vi "Actor Core.vi"(8 "error in":errorcluster, 11 "Example Actor in":refnum<class "Example Actor.lvclass">) -> (0 "error out":errorcluster, 3 "Actor out":refnum<class "Actor.lvclass">)   [LabVIEW 2023, in "Example Iterator NR Actor Implicit Iteration.lvlib" / "Example Actor.lvclass"]
doc: "(<B>Filename</B>: Actor Framework.lvlib:Actor.lvclass:Actor Core.vi)\n\nReceives messages to the actor, reacts to them, and initiates any error handling that may shut the actor down.\n\nDescendant classes may override this VI to append parallel tasks for the actor to complete while it handles messages. Overrides use the Call Parent Method node."
uses:
  Example Actor.lvclass
  <vilib>/ActorFramework/Actor/Actor.lvclass
  Iterator Settings.ctl
  Abstract Iterator Actor/Active Stop Conditions.ctl
  Abstract Iterator Actor/Stop Reason.ctl
  Iterator NR Actor/Iterator NR Actor Folder/Iterator NR Actor.lvclass
  Example Actor.lvclass/Example Actor.ctl
  <vilib>/ActorFramework/Actor/Actor.lvclass/Actor.ctl
  <vilib>/ActorFramework/Message Enqueuer/Message Enqueuer.lvclass/Message Enqueuer.ctl
  Example Actor Messages/Iterate Reply Msg/Iteration Msg.lvclass
  Abstract Iterator Actor/Iterator Settings.ctl
  <vilib>/ActorFramework/Message/Message.lvclass
  Iterator Actor/Iterator Actor Abstract Messages/Iterator Report Iterations End Msg/Iterator Report Iterations End Msg.lvclass
  <vilib>/ActorFramework/Message Enqueuer/Message Priority.ctl
  Example Actor Messages/Pre Iterate Reply Msg/Pre Iteration Msg.lvclass
  Example Actor Messages/Post Iterate Reply Msg/Post Iteration Msg.lvclass
  Example Actor Messages/Update Error Msg/Update Error Msg.lvclass
  <vilib>/ActorFramework/Message Enqueuer/Init from Existing Queue.vi
  <vilib>/ActorFramework/Message Enqueuer/Enqueue.vi
  <vilib>/ActorFramework/Stop Msg/Stop Msg.lvclass
  <vilib>/ActorFramework/Message Priority Queue/Priority Enqueue.vi
  <vilib>/ActorFramework/Message Enqueuer/Message Enqueuer.lvclass
  Example Actor Messages/Write Ready for iterations Msg/Write Ready for iterations Msg.lvclass
  Iterator Actor/Iterator Actor Messages/Write Settings Msg/Write Settings Msg.lvclass
  Iterator Actor/Iterator Actor Messages/Start Iterations Msg/Start Iterations Msg.lvclass
  Iterator Actor/Iterator Actor Messages/Stop Iterations Msg/Stop Iterations Msg.lvclass
  C:/Program Files/National Instruments/LabVIEW 2023/vi.lib/ActorFramework/Actor/Actor.lvclass
  C:/Projects/Iterator Actor/Examples/Example Iterator NR Actor Implicit Iteration/Example Actor/Example Actor.lvclass
  Abstract Iterator Actor/Abstract Iterator Actor.lvclass
  C:/Projects/Iterator Actor/Abstract Iterator Actor/Abstract Iterator Actor.lvclass
  C:/Program Files/National Instruments/LabVIEW 2023/vi.lib/LS Instruments AG/Async Methods Actor/Async Methods Actor/Async Methods Actor/Async Methods Actor.lvclass
  C:/Projects/Iterator Actor/Iterator NR Actor/Iterator NR Actor Folder/Iterator NR Actor.lvclass
  C:/Projects/Iterator Actor/Iterator NR Actor/Iterator NR Actor Messages/Iteration Msg/Abstract Iteration Msg.lvclass
  C:/Program Files/National Instruments/LabVIEW 2023/vi.lib/ActorFramework/Message/Message.lvclass
  C:/Projects/Iterator Actor/Examples/Example Iterator NR Actor Implicit Iteration/Example Actor Messages/Iterate Reply Msg/Iteration Msg.lvclass
  C:/Projects/Iterator Actor/Examples/Example Iterator NR Actor Implicit Iteration/Example Actor Messages/Pre Iterate Reply Msg/Pre Iteration Msg.lvclass
  C:/Projects/Iterator Actor/Examples/Example Iterator NR Actor Implicit Iteration/Example Actor Messages/Post Iterate Reply Msg/Post Iteration Msg.lvclass
  C:/Projects/Iterator Actor/Iterator Actor/Iterator Actor Abstract Messages/Iterator Report Iterations End Msg/Iterator Report Iterations End Msg.lvclass
  C:/Projects/Iterator Actor/Examples/Example Iterator NR Actor Implicit Iteration/Example Actor Messages/Update Error Msg/Update Error Msg.lvclass
panel:
  out "Stop Reason":T1
  in  "Receive report":bool=TRUE
  in  "Do post-iterations":bool=TRUE
  in  "Do pre-iterations":bool=TRUE
  out "Iterator error":errorcluster
  in  "User Settings":T2={"Prepare timeout (ms)"=1000, "Iterate timeout (ms)"=1000, "Conclude timeout (ms)"=1000, "Iterate period (ms)"=1000, "Active Stop Conditions"={"Number of Iterations"=FALSE, "Time Elapsed"=FALSE, "Iteration Result"=FALSE}, "Iterations"=5, "Time before stop (ms)"=200}
  out "Post Iterate":bool
  out "Pre Iterate":bool
  in  "exit":bool
  out "Iterate":bool
  in  "stop iterations":bool
  in  "start iterations":bool
  in  "Ready for iterations":bool=TRUE
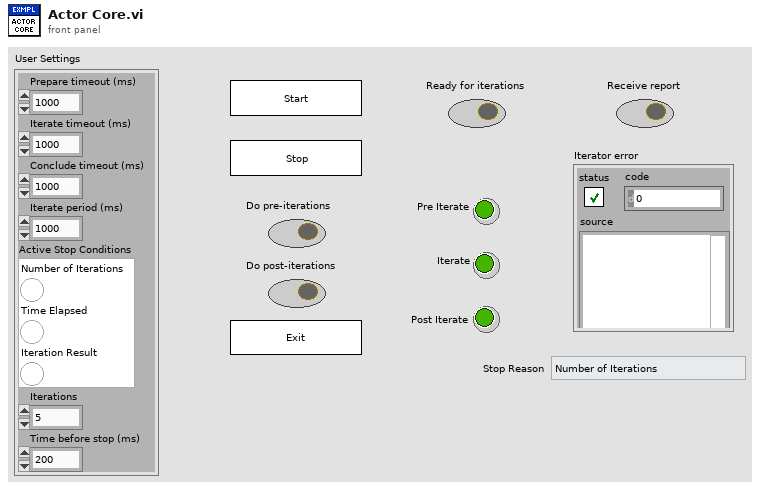
[diagram p1: front panel]
types:
  T1 = typedef "Iterator Actor.lvlib/Abstract Iterator Actor.lvclass/Stop Reason.ctl" = enum16{"Number of Iterations", "Time Elapsed", "Stopped Internally", "Stopped Externally"}
  T2 = typedef "Example Iterator NR Actor Implicit Iteration.lvlib/Example Actor.lvclass/Iterator Settings.ctl" = cluster{"Prepare timeout (ms)":i32, "Iterate timeout (ms)":i32, "Conclude timeout (ms)":i32, "Iterate period (ms)":i32, "Active Stop Conditions":T3, "Iterations":i32, "Time before stop (ms)":i32}
  T3 = typedef "Iterator Actor.lvlib/Abstract Iterator Actor.lvclass/Active Stop Conditions.ctl" = cluster{"Number of Iterations":bool, "Time Elapsed":bool, "Iteration Result":bool}
  T4 = typedef "Iterator Actor.lvlib/Abstract Iterator Actor.lvclass/Iterator Settings.ctl" = cluster{"Prepare timeout (ms)":i32, "Iterate timeout (ms)":i32, "Conclude timeout (ms)":i32, "Iterate period (ms)":i32, "Number of iterations":i32, "Time before stop (ms)":i32, "Active Stop Conditions":T3, "Prepare Msg":refnum<class "Message.lvclass">, "Iterate Msg":refnum<class "Message.lvclass">, "Conclude Msg":refnum<class "Message.lvclass">, "Iterations End Report":refnum<class "Iterator Report Iterations End Msg.lvclass">, "Message Priority (Normal)":T5}
  T5 = typedef "Actor Framework.lvlib/Message Enqueuer.lvclass/Message Priority.ctl" = enum16{"Low", "Normal", "High"}
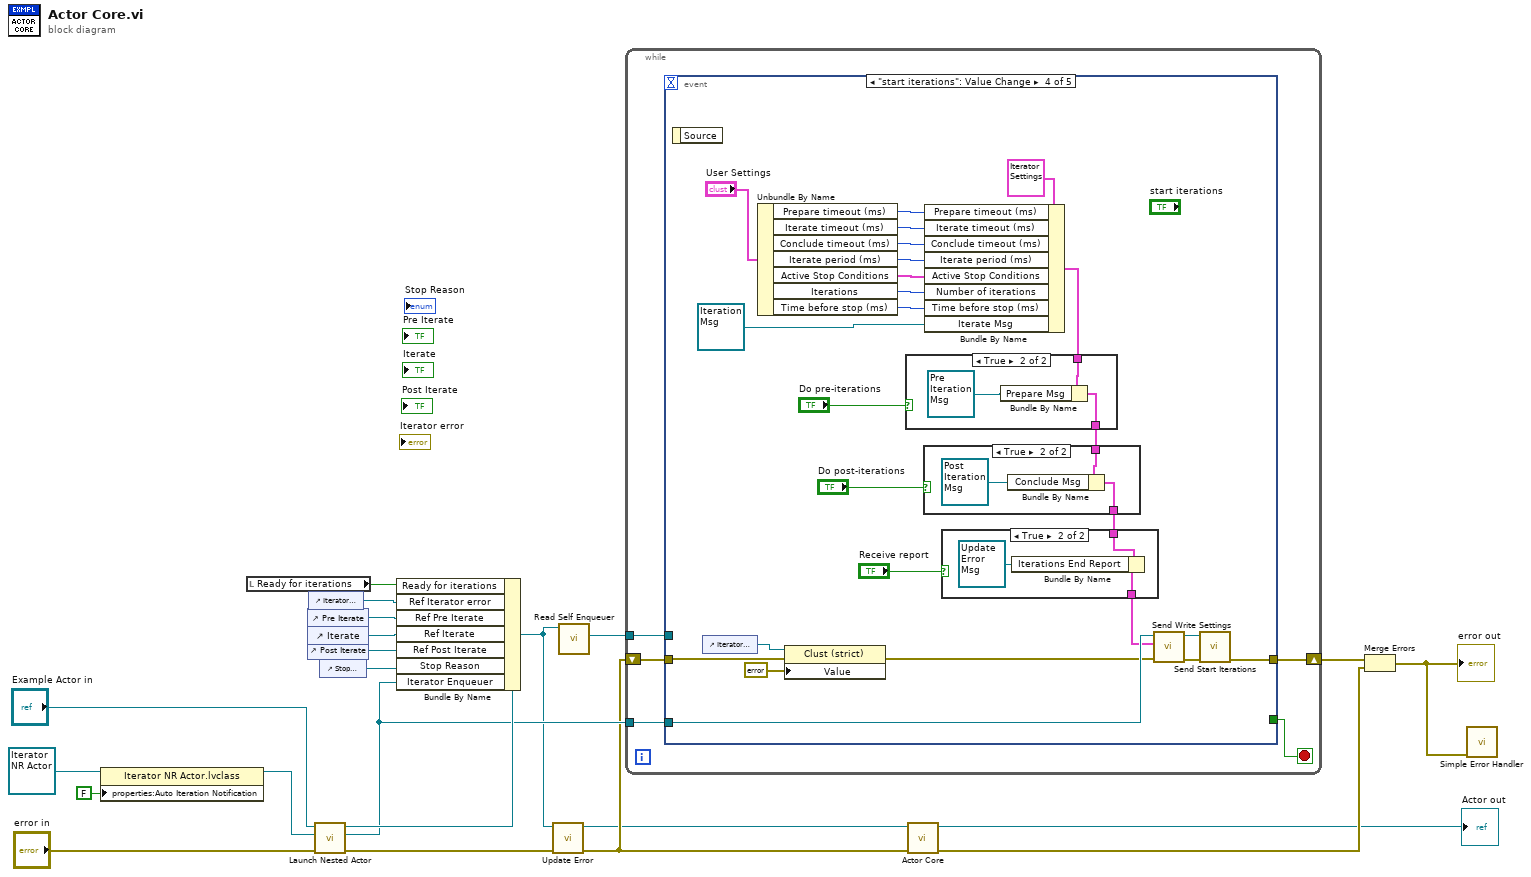
[diagram p0: block diagram]
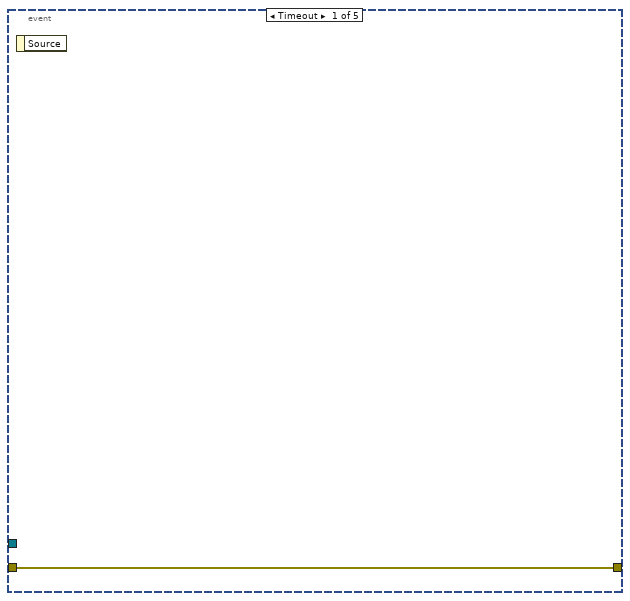
[diagram p2: hidden frame]
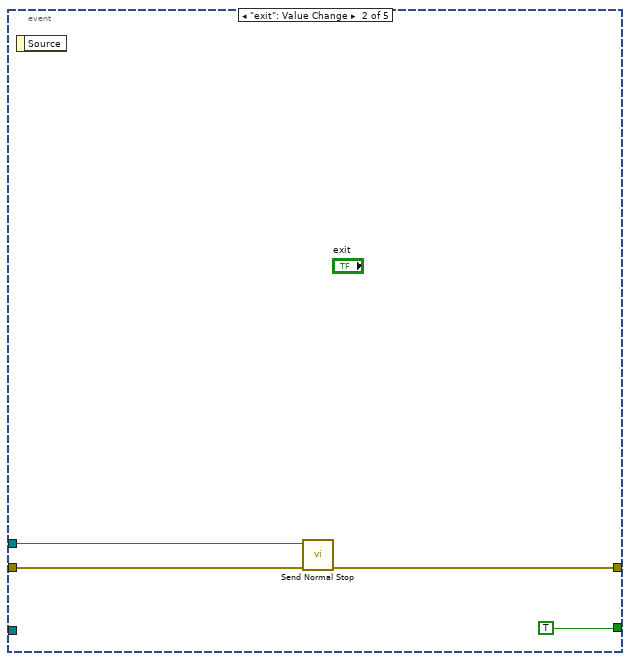
[diagram p3: hidden frame]
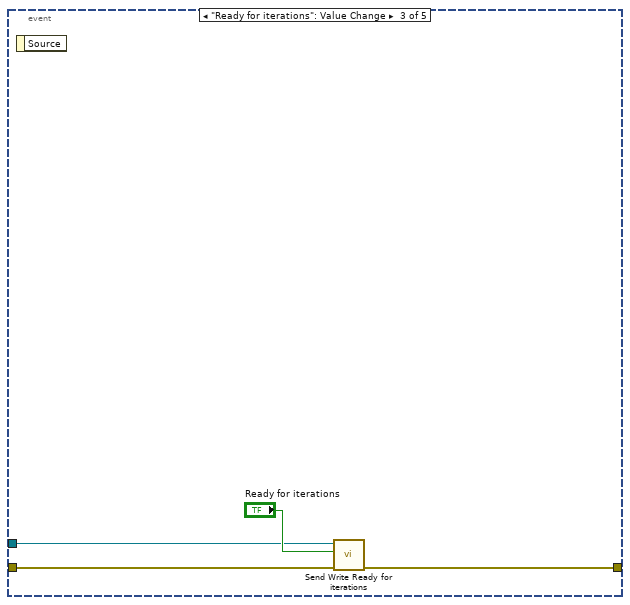
[diagram p4: hidden frame]
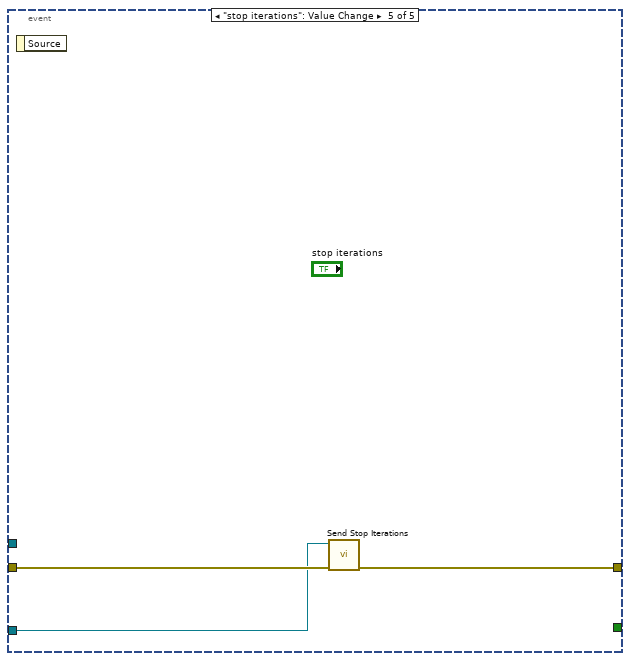
[diagram p8: hidden frame]
diagram:
  n1 = property class="Iterator NR Actor.lvclass"(reference=refnum<class "Iterator NR Actor.lvclass"> refnum ("Iterator Actor 2.lvlib:Iterator Actor 2.lvclass"), "properties:Auto Iteration Notification"=FALSE ("Auto Iteration Notification")) -> (reference out=w2:refnum<class "Iterator NR Actor.lvclass">)  [unwired: 1 in, 1 out]
  n2 = local read "Ready for iterations"() -> (w13:bool)
  n3 = control-ref of="Pre Iterate"() -> (w18:refnum<vi>)
  n4 = control-ref of="Iterate"() -> (w17:refnum<vi>)
  n5 = control-ref of="Post Iterate"() -> (w16:refnum<vi>)
  n6 = control-ref of="Iterator error"() -> (w11:refnum<vi>)
  n7 = call <vilib>:"Launch Nested Actor.vi"("error in (no error)"="error in", "Nested Actor"=w2, "Caller Actor in"="Example Actor in") -> ("error out"=w10:errorcluster, "Nested Actor's Enqueuer"=w14:refnum<class "Message Enqueuer.lvclass">, "Caller Actor out"=w15:refnum<class "Example Actor.lvclass">)  [unwired: 6 in]
  n8 = control-ref of="Stop Reason"() -> (w6:refnum<vi>)
  n9 = Bundle By Name(cluster=w15, "Ready for iterations"=w13, "Ref Iterator error"=w11, "Ref Pre Iterate"=w18, "Ref Iterate"=w17, "Ref Post Iterate"=w16, "Stop Reason"=w6, "Iterator Enqueuer"=w14) -> (w8:refnum<class "Example Actor.lvclass">)
  n10 = call "Update Error.vi"("error in (no error)"=w10, "Example Actor in"=w8) -> ("error out"=w9:errorcluster, "Example Actor out"=w7:refnum<class "Example Actor.lvclass">)  [unwired: 8 in]
  n11 = call <vilib>:"Read Self Enqueuer.vi"("Actor"=w8) -> ("Self Enqueuer"=w22:refnum<class "Message Enqueuer.lvclass">)  [unwired: 10 in]
  n12 = while {
    tunnel: w22 -> [w27]
    shift-right: [w26] -> w21
    shift-left: w9 -> [w25]
    tunnel: w14 -> [w23]
    stop <- w24 stop-if-true
    n13 = event shown="[3] \"start iterations\": Value Change" {
      selector: _ -> [_ _ _ _ _]
      dyn-events: _ -> [_ _ _ _ _]
      timeout: _ -> [_ _ _ _ _]
      tunnel: w27 -> [_ w32 w33 _ _]
      tunnel: [w28 w31 w34 w46 w75] -> w26
      tunnel: w25 -> [w28 w30 w36 w49 w76]
      tunnel: [_ TRUE _ _ _] -> w24
      tunnel: w23 -> [_ _ _ w60 w74]
      event Timeout {
        n14 = event-data() -> ()  [unwired: 1 in, 1 out]
      }
      event "exit": Value Change {
        n15 = event-data() -> ()  [unwired: 1 in, 1 out]
        n16 = call <vilib>:"Send Normal Stop.vi"("error in (no error)"=w30, "Message Enqueuer"=w32) -> ("error out"=w31:errorcluster)  [unwired: 9 in]
      }
      event "Ready for iterations": Value Change {
        n17 = event-data() -> ()  [unwired: 1 in, 1 out]
        n18 = call "Send Write Ready for iterations.vi"("error in (no error)"=w36, "Ready for iterations"="Ready for iterations", "Message Enqueuer in"=w33) -> ("error out"=w34:errorcluster)  [unwired: 7 in, 1 out]
      }
      event "start iterations": Value Change {
        n19 = event-data() -> ()  [unwired: 1 in, 1 out]
        n20 = control-ref of="Iterator error"() -> (w48:refnum<vi>)
        n21 = Unbundle By Name("User Settings") -> ("Prepare timeout (ms)"=w53:i32, "Iterate timeout (ms)"=w54:i32, "Conclude timeout (ms)"=w55:i32, "Iterate period (ms)"=w56:i32, "Active Stop Conditions"=w50:T3, "Iterations"=w51:i32, "Time before stop (ms)"=w52:i32)
        n22 = property class="Clust (strict)"(reference=w48, error in=w49, "Value"=errorcluster {"status"=FALSE, "code"=0, "source"=""}) -> (error out=w44:errorcluster)  [unwired: 1 out]
        n23 = Bundle By Name(cluster=T4 {"Prepare timeout (ms)"=0, "Iterate timeout (ms)"=0, "Conclude timeout (ms)"=0, "Iterate period (ms)"=0, "Number of iterations"=0, "Time before stop (ms)"=0, "Active Stop Conditions"={"Number of Iterations"=FALSE, "Time Elapsed"=FALSE, "Iteration Result"=FALSE}, "Prepare Msg"=refnum, "Iterate Msg"=refnum, "Conclude Msg"=refnum, "Iterations End Report"=refnum, "Message Priority (Normal)"=enum."Normal"} ("Iterator Settings"), "Prepare timeout (ms)"=w53, "Iterate timeout (ms)"=w54, "Conclude timeout (ms)"=w55, "Iterate period (ms)"=w56, "Active Stop Conditions"=w50, "Number of iterations"=w51, "Time before stop (ms)"=w52, "Iterate Msg"=refnum<class "Iteration Msg.lvclass"> refnum ("Example Actor.lvlib:Iterate Reply Msg.lvclass")) -> (w41:T4)
        n24 = case shown="True" "Do pre-iterations" {
          tunnel: w41 -> [w70 w73]
          tunnel: [w70 w71] -> w40
          frame False {
          }
          frame True {
            n25 = Bundle By Name(cluster=w73, "Prepare Msg"=refnum<class "Pre Iteration Msg.lvclass"> refnum ("Example Actor.lvlib:Pre Iterate Reply Msg.lvclass")) -> (w71:T4)
          }
        }
        n26 = case shown="True" "Do post-iterations" {
          tunnel: w40 -> [w66 w69]
          tunnel: [w66 w67] -> w38
          frame False {
          }
          frame True {
            n27 = Bundle By Name(cluster=w69, "Conclude Msg"=refnum<class "Post Iteration Msg.lvclass"> refnum ("Example Actor.lvlib:Post Iterate Reply Msg.lvclass")) -> (w67:T4)
          }
        }
        n28 = case shown="True" "Receive report" {
          tunnel: [w62 w65] -> w37
          tunnel: w38 -> [w62 w64]
          frame False {
          }
          frame True {
            n29 = Bundle By Name(cluster=w64, "Iterations End Report"=refnum<class "Update Error Msg.lvclass"> refnum ("Example Actor.lvlib:Update Error Msg.lvclass")) -> (w65:T4)
          }
        }
        n30 = call "Send Write Settings.vi"("error in (no error)"=w44, "Settings"=w37, "Message Enqueuer in"=w60) -> ("error out"=w61:errorcluster, "Message Enqueuer out"=w45:refnum<class "Message Enqueuer.lvclass">)  [unwired: 7 in]
        n31 = call "Send Start Iterations.vi"("error in (no error)"=w61, "Message Enqueuer in"=w45) -> ("error out"=w46:errorcluster)  [unwired: 8 in, 1 out]
      }
      event "stop iterations": Value Change {
        n32 = event-data() -> ()  [unwired: 1 in, 1 out]
        n33 = call "Send Stop Iterations.vi"("error in (no error)"=w76, "Message Enqueuer in"=w74) -> ("error out"=w75:errorcluster)  [unwired: 8 in, 1 out]
      }
    }
  }
  n34 = call-parent "Actor Core.vi"("error in"=w9, "Actor in"=w7) -> ("error out"=w20:errorcluster, "Actor out"=→"Actor out":refnum<class "Actor.lvclass">)  [unwired: 8 in]
  n35 = Merge Errors(w21, w20) -> (w12:errorcluster)
  "error out" <- w12
  n36 = call <vilib>:"Simple Error Handler.vi"("error in (no error)"=w12) -> ()  [unwired: 4 in, 5 out]
